vi "Handle Command.vi"(8 "error in (no error)":errorcluster, 9 "Data":variant, 10 "Command":string, 11 "Inst.MOTOR in":refnum<class "Inst.MOTOR.lvclass">) -> (0 "error out":errorcluster, 1 "Processed Data":variant, 2 "Command":string, 3 "Inst.MOTOR out":refnum<class "Inst.MOTOR.lvclass">)   [LabVIEW 2019, in "Inst.MOTOR.lvclass"]
uses:
  Inst.MOTOR.lvclass
  Typedefs/Inst.MOTOR.getAll--Cluster.ctl
  Inst.MOTOR.lvclass/Inst.MOTOR.ctl
  9aec49fd-fe04-463a-be35-b7075f22e824.vi
  9aec49fd-fe04-463a-be35-b7075f22e824.vi/78140b32-a3ea-4794-a7df-724a2863ea3d.vi
  9aec49fd-fe04-463a-be35-b7075f22e824.vi/bca7f9cd-eb60-4417-b9ac-5471ad6f13ca.vi
  <vilib>/Utility/Data Type/Get Type Information.vi
  <vilib>/JDP Science/JSONtext/JSON text to Variant.vi
  <vilib>/JDP Science/JSONtext/LVClass Serializer/JSONtext LVClass Serializer.lvclass
  <userlib>/LevyLab/Instrument Framework/Instrument Types/VSource/Instrument.VSource.lvclass
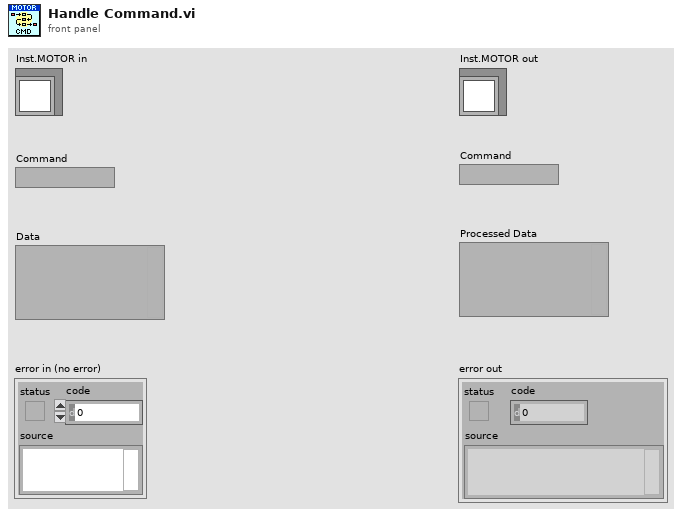
[diagram p1: front panel]
types:
  T1 = typedef "Inst.MOTOR.lvclass/Inst.MOTOR.getAll--Cluster.ctl" = cluster{"Response":string, "Forward":bool, "Stop Motor":bool, "Encoder Position":string}
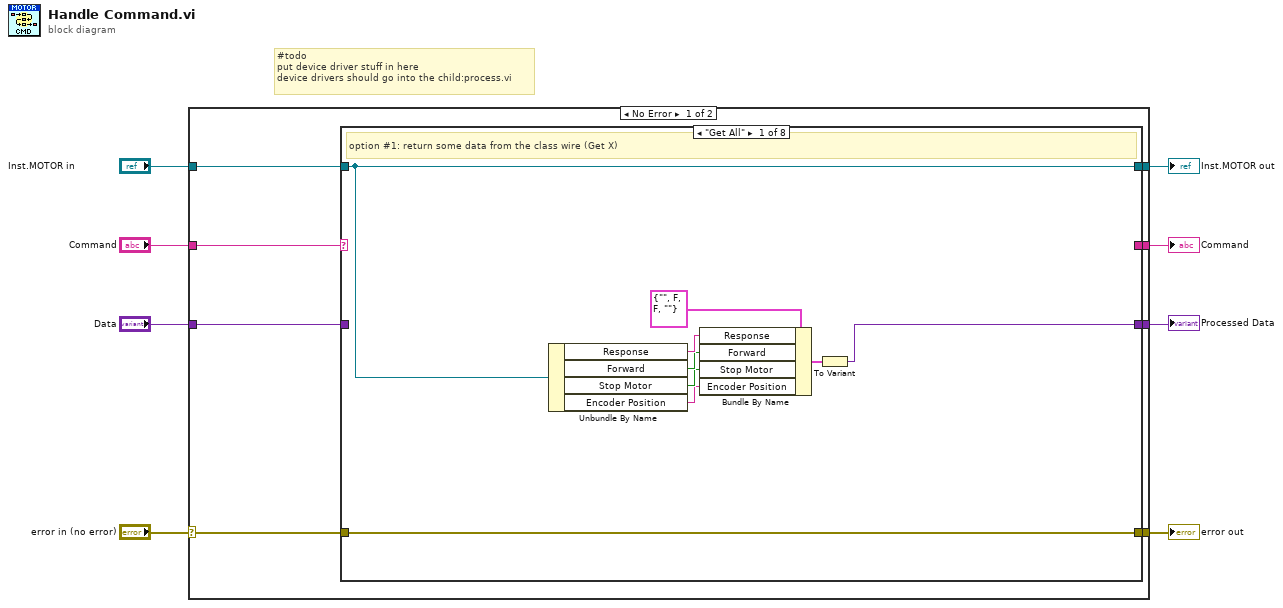
[diagram p0: block diagram]
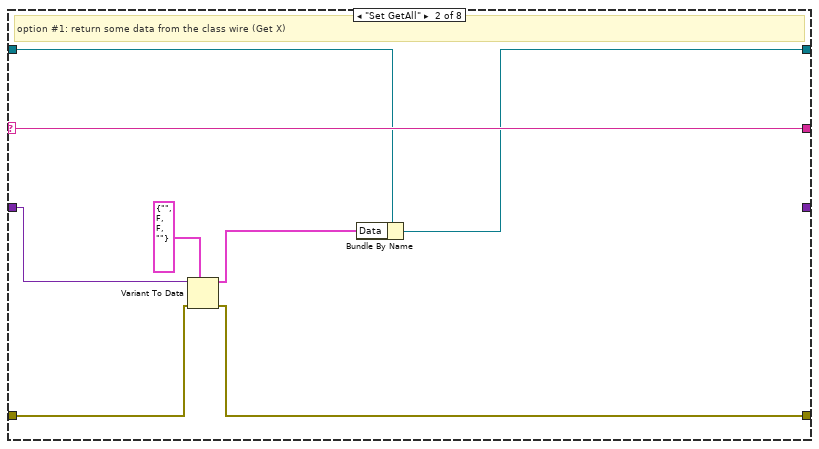
[diagram p2: hidden frame]
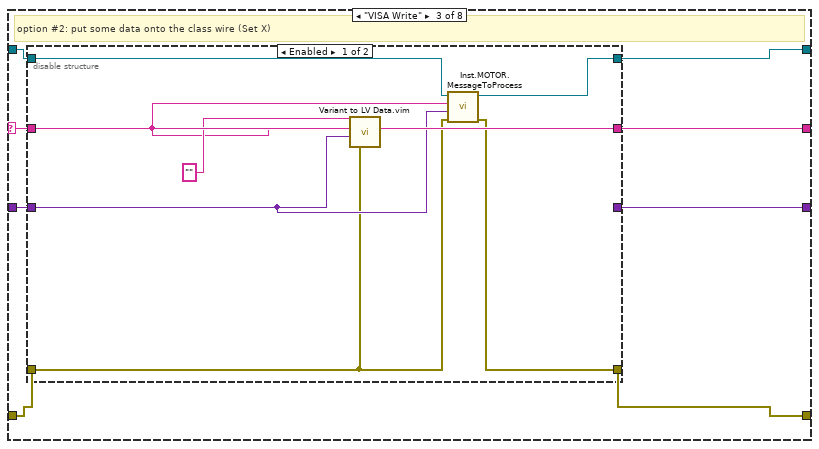
[diagram p3: hidden frame]
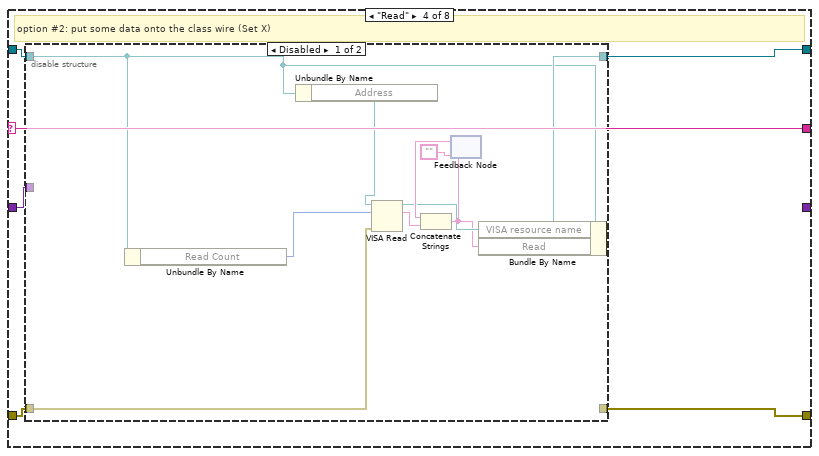
[diagram p5: hidden frame]
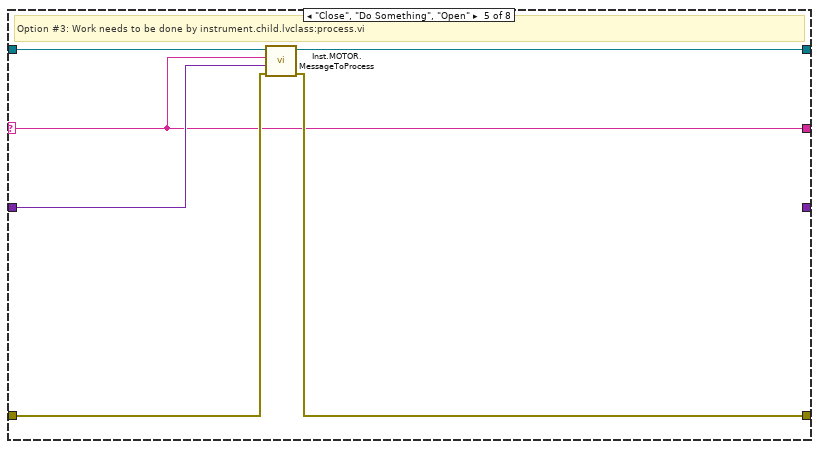
[diagram p7: hidden frame]
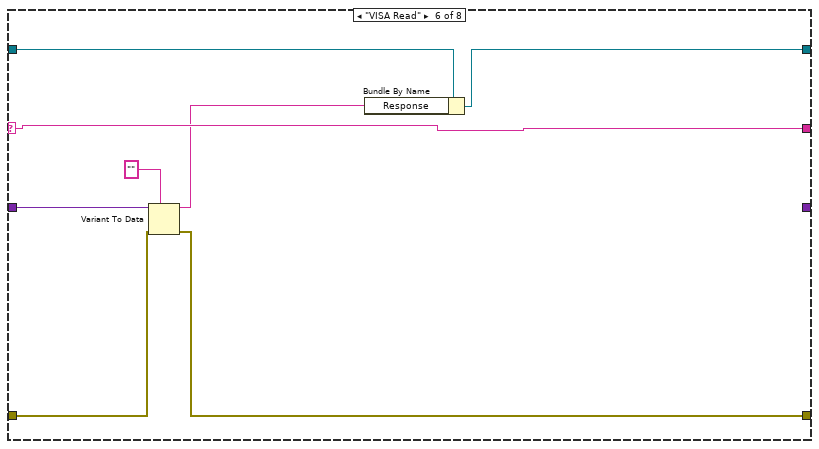
[diagram p8: hidden frame]
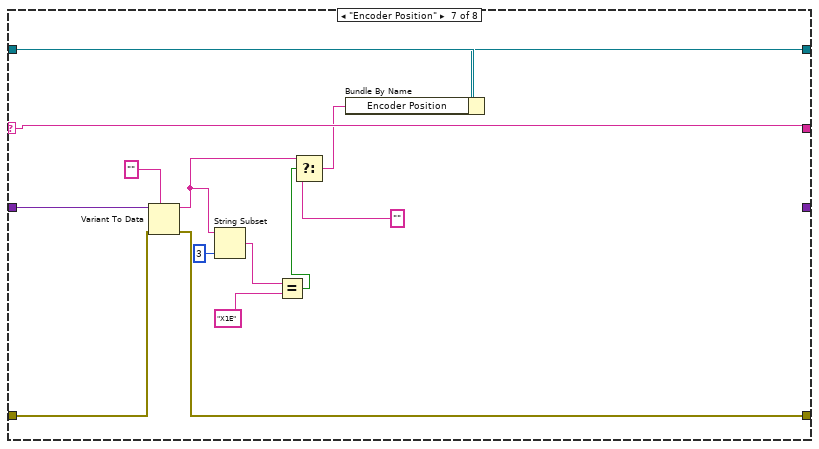
[diagram p9: hidden frame]
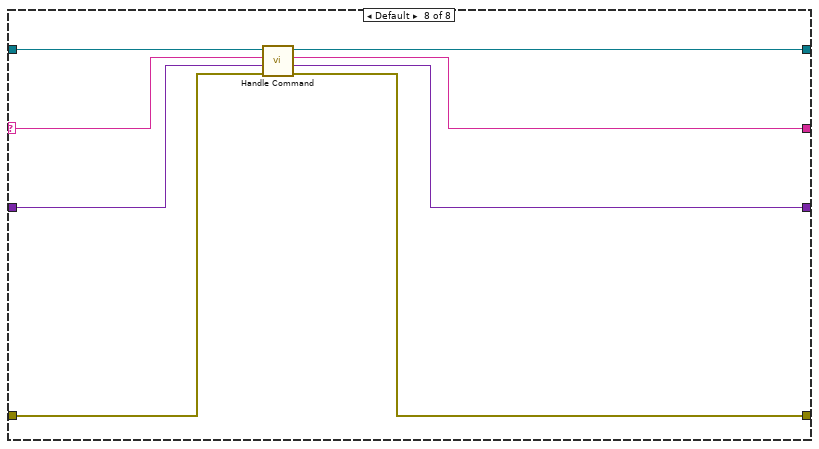
[diagram p10: hidden frame]
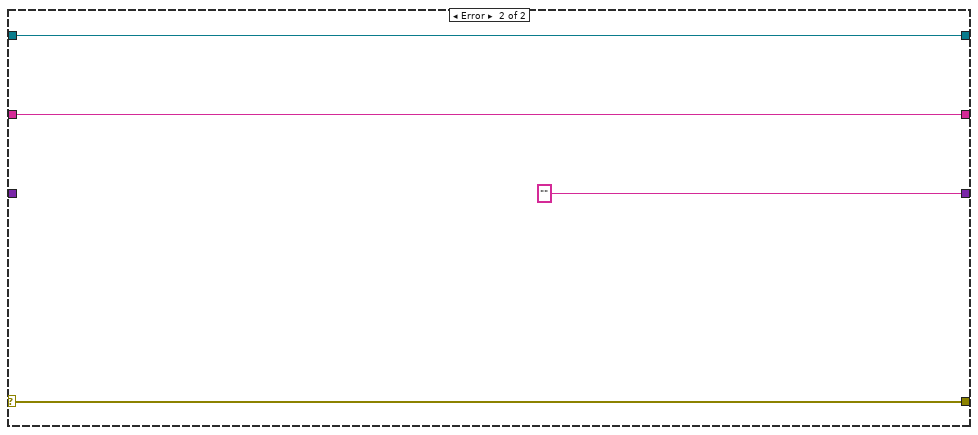
[diagram p11: hidden frame]
diagram:
  # "#todo\nput device driver stuff in here\ndevice drivers should go into the child:process.vi"
  n1 = case shown="No Error" "error in (no error)" {
    selector: "error in (no error)" -> [w10 w110]
    tunnel: [w12 w110] -> w6
    tunnel: [w14 w109] -> w5
    tunnel: "Inst.MOTOR in" -> [w15 w109]
    tunnel: "Command" -> [w16 w107]
    tunnel: [w13 "" ("String")] -> w3
    tunnel: "Data" -> [w9 _]
    tunnel: [w11 w107] -> w1
    frame No Error {
      n2 = case shown="\"Get All\"" w16 {
        selector: w16 -> [_ w33 w34 w52 w71 w84 w98 w100]
        tunnel: w15 -> [w23 w27 w36 w53 w76 w83 w97 w104]
        tunnel: [w23 w28 w40 w56 w75 w77 w92 w101] -> w14
        tunnel: [w24 _ w35 _ _ _ _ w103] -> w13
        tunnel: w10 -> [w25 w26 w39 w54 w74 w78 w93 w105]
        tunnel: w9 -> [_ w32 w38 w51 w72 w82 w96 w106]
        tunnel: [w25 w31 w37 w55 w73 w79 w94 w102] -> w12
        tunnel: [_ w33 w34 w52 w71 w84 w98 w99] -> w11
        frame "Get All" {
          # "option #1: return some data from the class wire (Get X)"
          n3 = Unbundle By Name(w23) -> ("Response"=w20:string, "Forward"=w19:bool, "Stop Motor"=w18:bool, "Encoder Position"=w17:string)
          n4 = Bundle By Name(cluster=T1 {"Response"="", "Forward"=FALSE, "Stop Motor"=FALSE, "Encoder Position"=""} ("getAll"), "Response"=w20, "Forward"=w19, "Stop Motor"=w18, "Encoder Position"=w17) -> (w21:T1)
          n5 = To Variant(anything=w21) -> (Variant=w24:variant)
        }
        frame "Set GetAll" {
          # "option #1: return some data from the class wire (Get X)"
          n6 = Variant To Data(error in=w26, type=T1 {"Response"="", "Forward"=FALSE, "Stop Motor"=FALSE, "Encoder Position"=""} ("getAll"), Variant=w32) -> (data=w29:T1, error out=w31:errorcluster)
          n7 = Bundle By Name(cluster=w27, "Data"=w29) -> (w28:refnum<class "Inst.MOTOR.lvclass">)
        }
        frame "VISA Write" {
          # "option #2: put some data onto the class wire (Set X)"
          n8 = disable-structure shown="Enabled" {
            disable-tunnel: [w45 w50] -> w40
            disable-tunnel: w39 -> [w42 w48]
            disable-tunnel: w38 -> [w43 w49]
            disable-tunnel: w34 -> [w44 _]
            disable-tunnel: [w41 w48] -> w37
            disable-tunnel: w36 -> [w46 w50]
            disable-tunnel: [_ w49] -> w35
            disable-tunnel: w34 -> [_ _]
            frame Enabled {
              n9 = call "Variant to LV Data.vim"("type"="", "error in (no error)"=w42, "JSON Data in"=w43, "Command"=w44) -> ()  [unwired: 4 in, 4 out]
              n10 = call "Inst.MOTOR.MessageToProcess.vi"("error in (no error)"=w42, "Data"=w43, "Command"=w44, "Inst.MOTOR in"=w46) -> ("error out"=w41:errorcluster, "Inst.MOTOR out"=w45:refnum<class "Inst.MOTOR.lvclass">)  [unwired: 6 in]
            }
            frame Disabled {
            }
          }
        }
        frame "Read" {
          # "option #2: put some data onto the class wire (Set X)"
          n11 = disable-structure shown="Disabled" {
            disable-tunnel: [w68 w70] -> w56
            disable-tunnel: [w58 w69] -> w55
            disable-tunnel: w54 -> [w63 w69]
            disable-tunnel: w53 -> [w61 w70]
            disable-tunnel: w51 -> [_ _]
            frame Disabled {
              n12 = Unbundle By Name(w61) -> ("Read Count"=w62:u32)
              n13 = Unbundle By Name(w61) -> ("Address"=w67:refnum<visa-resource-name>)
              n14 = VISA Read(VISA resource name=w67, byte count=w62, error in (no error)=w63) -> (VISA resource name out=w60:refnum<visa-resource-name>, read buffer=w65:string, error out=w59:errorcluster)  [unwired: 1 out]
              n15 = feedback #1("") -> (w64:string)
              n16 = Concatenate Strings(w64, w65) -> (w57:string)
              n17 = feedback-in #1(w57) -> ()
              n18 = Bundle By Name(cluster=w61, "VISA resource name"=w60, "Read"=w57) -> (w68:refnum<class "Inst.MOTOR.lvclass">)
            }
            frame Enabled {
            }
          }
        }
        frame "Close", "Do Something", "Open" {
          # "Option #3: Work needs to be done by instrument.child.lvclass:process.vi"
          n19 = call "Inst.MOTOR.MessageToProcess.vi"("error in (no error)"=w74, "Data"=w72, "Command"=w71, "Inst.MOTOR in"=w76) -> ("error out"=w73:errorcluster, "Inst.MOTOR out"=w75:refnum<class "Inst.MOTOR.lvclass">)  [unwired: 6 in]
        }
        frame "VISA Read" {
          n20 = Variant To Data(error in=w78, type="", Variant=w82) -> (data=w80:string, error out=w79:errorcluster)
          n21 = Bundle By Name(cluster=w83, "Response"=w80) -> (w77:refnum<class "Inst.MOTOR.lvclass">)
        }
        frame "Encoder Position" {
          n22 = Variant To Data(error in=w93, type="", Variant=w96) -> (data=w87:string, error out=w94:errorcluster)
          n23 = String Subset(string=w87, length (rest)=3 ("length (rest)")) -> (substring=w85:string)  [unwired: 1 in]
          n24 = Equal?(x=w85, y="X1E") -> (x = y?=w89:bool)
          n25 = Select(t=w87, s=w89, f="") -> (s? t:f=w90:string)
          n26 = Bundle By Name(cluster=w97, "Encoder Position"=w90) -> (w92:refnum<class "Inst.MOTOR.lvclass">)
        }
        frame Default {
          n27 = call-parent "Handle Command.vi"("error in (no error)"=w105, "Data"=w106, "Command"=w100, "Instrument in"=w104) -> ("error out"=w102:errorcluster, "Processed Data"=w103:variant, "Command"=w99:string, "Instrument out"=w101:refnum<class "Inst.MOTOR.lvclass">)  [unwired: 4 in]
        }
      }
    }
    frame Error {
    }
  }
  "error out" <- w6
  "Inst.MOTOR out" <- w5
  "Command" <- w1
  "Processed Data" <- w3
